vi "Query Relay State.vi"(8 "error in":errorcluster, 11 "2575 in":refnum<class "2575.lvclass">) -> (0 "error out":errorcluster, 2 "Relay State":bool[](array[boolean]), 3 "2575 out":refnum<class "2575.lvclass">)   [LabVIEW 2019, in "2575.lvlib" / "2575.lvclass"]
uses:
  Library/2575.lvclass
  C:/Users/Public/Documents/Development/builds/Instruments/SwitchMatrix.lvlibp/SwitchMatrix.lvclass
  Library/2575.lvclass/2575.ctl
  <instrlib>/niSwitch/niSwitch.llb/niSwitch Relay Position.ctl
  Accessors/Read Local Resource.vi
  Accessors/Read Device Relay Name.vi
  Accessors/Read Relay Map.vi
  Accessors/Write Local Resource.vi
  builds/Instruments/SwitchMatrix.lvlibp/Accessors/Write Relay State.vi
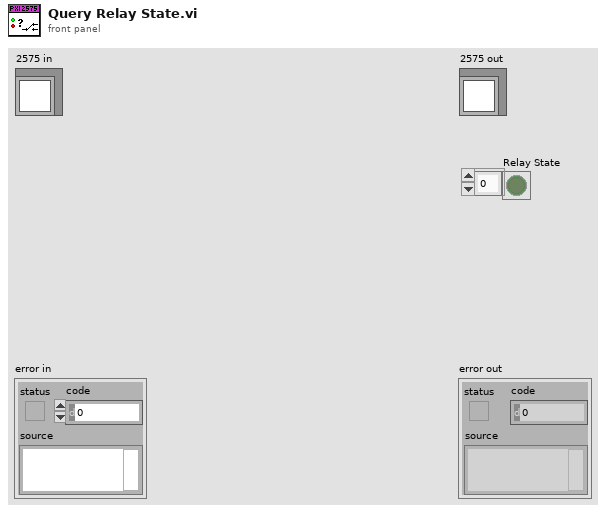
[diagram p1: front panel]
types:
  T1 = typedef "niSwitch Relay Position.ctl" = i32
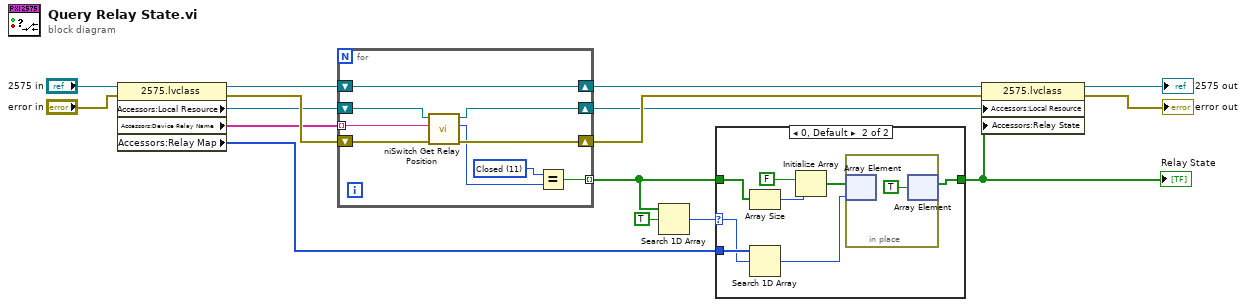
[diagram p0: block diagram]
diagram:
  n1 = property class="2575.lvclass"(reference="2575 in", error in="error in") -> (reference out=w11:refnum<class "2575.lvclass">, error out=w16:errorcluster, "Accessors:Local Resource"=w9:refnum<k15>, "Accessors:Device Relay Name"=w10:string[], "Accessors:Relay Map"=w7:i32[])
  n2 = for {
    shift-right: [w25] -> w5
    shift-left: w11 -> [w25]
    shift-right: [w20] -> w6
    shift-left: w16 -> [w22]
    shift-right: [w21] -> w4
    shift-left: w9 -> [w24]
    tunnel: w10 -> [w23] mode=indexing
    tunnel: [w17] -> w2 mode=indexing
    w18 = T1 11 items=["Open"=10, "Closed"=11] ("x")
    n3 = call <instrlib>:"niSwitch Get Relay Position.vi"("error in (no error)"=w22, "relay name"=w23, "instrument handle"=w24) -> ("error out"=w20:errorcluster, "position"=w19:T1, "instrument handle out"=w21:refnum<k15>)  [unwired: 6 in]
    n4 = Equal?(x=w18, y=w19) -> (x = y?=w17:bool)
  }
  n5 = Search 1D Array(1D array=w2, element=TRUE) -> (index of element=w3:i32)  [unwired: 1 in]
  n6 = case shown="0, Default" w3 {
    selector: w3 -> [_ w33]
    tunnel: w2 -> [w26 w32]
    tunnel: [w26 w28] -> w8
    tunnel: w7 -> [_ w34]
    frame -1 {
    }
    frame 0, Default {
      n7 = Array Size(array=w32) -> (size(s)=w31:i32)
      n8 = Search 1D Array(1D array=w34, element=w33) -> (index of element=w27:i32)  [unwired: 1 in]
      n9 = Initialize Array(FALSE, w31) -> (w29:bool[])
      n10 = in-place {
        n11 = in-place-array #1(w29, w27) -> ()  [unwired: 1 out]
        n12 = in-place-array #1(TRUE ("element")) -> (w28:bool[])  [unwired: 1 out]
      }
    }
  }
  "Relay State" <- w8
  n13 = property class="2575.lvclass"(reference=w5, error in=w6, "Accessors:Local Resource"=w4, "Accessors:Relay State"=w8) -> (reference out=→"2575 out":refnum<class "2575.lvclass">, error out=→"error out":errorcluster)
